vi "Get N Images.vi"(8 "error in":errorcluster, 10 "count (-1 = all)":i32=-1, 11 "Worker in":refnum<class "Camera Worker.lvclass">) -> (0 "error out":errorcluster, 2 "IImages":refnum<class "Generic Image.lvclass">[](array[class]), 3 "Worker out":refnum<class "Camera Worker.lvclass">)   [LabVIEW 2025, in "Camera Worker.lvlib" / "Camera Worker.lvclass"]
uses:
  Camera Worker.lvclass
  Typedefs/Generic Image/Generic Image.lvclass
  Camera Worker.lvclass/Camera Worker.ctl
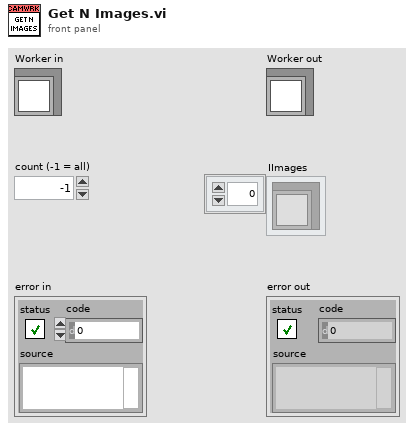
[diagram p1: front panel]
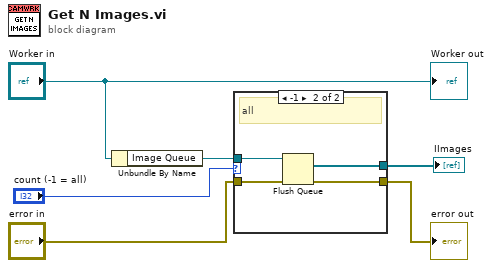
[diagram p0: block diagram]
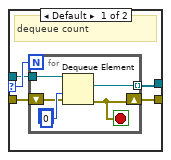
[diagram p2: hidden frame]
diagram:
  n1 = Unbundle By Name("Worker in") -> ("Image Queue"=w5:refnum<queue>)
  n2 = case shown="-1" "count (-1 = all)" {
    selector: "count (-1 = all)" -> [w11 _]
    tunnel: w5 -> [w10 w20]
    tunnel: "error in" -> [w7 w19]
    tunnel: [w8 w18] -> w3
    tunnel: [w9 w17] -> w1
    frame Default {
      # "dequeue count"
      n3 = for {
        N: w11 -> [_]
        tunnel: w10 -> [w16]
        tunnel: [w14] -> w9 mode=indexing
        shift-right: [w13] -> w8
        shift-left: w7 -> [w12]
        stop <- w13 stop-if-true
        n4 = Dequeue Element(queue=w16, timeout in ms (-1)=0, error in (no error)=w12) -> (element=w14:refnum<class "Generic Image.lvclass">, error out=w13:errorcluster)  [unwired: 2 out]
      }
    }
    frame -1 {
      # "all"
      n5 = Flush Queue(queue=w20, error in (no error)=w19) -> (remaining elements=w17:refnum<class "Generic Image.lvclass">[], error out=w18:errorcluster)  [unwired: 1 out]
    }
  }
  "error out" <- w3
  "IImages" <- w1
  "Worker out" <- "Worker in"
